vi "Edge Focus.vi"(8 "error in":errorcluster, 9 "Increment Size":dbl=-0.1 format="%#_13g", 10 "Position In":dbl=1.0 format="%#_13g", 11 "Gantry In":refnum<k24>) -> (0 "error out":errorcluster, 3 "Gantry Out":refnum<k24>)   [LabVIEW 2021, in "Component Tray.lvclass"]
uses:
  Component/Component Tray.lvclass
  C:/Program Files (x86)/Aerotech/A3200/LabVIEW/2010/Bin/Aerotech.A3200.dll
  Program Files (x86)/Aerotech/A3200/LabVIEW/2010/Bin/Aerotech.A3200.dll
  Controller/Motion/A3200/A3200.lvclass
  <vilib>/Analysis/NI_AALBase.lvlib
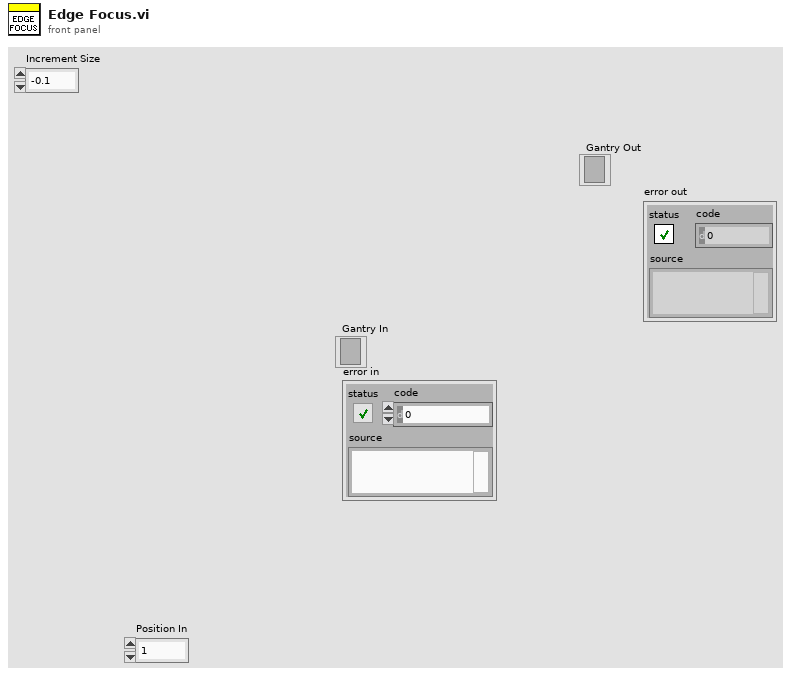
[diagram p1: front panel]
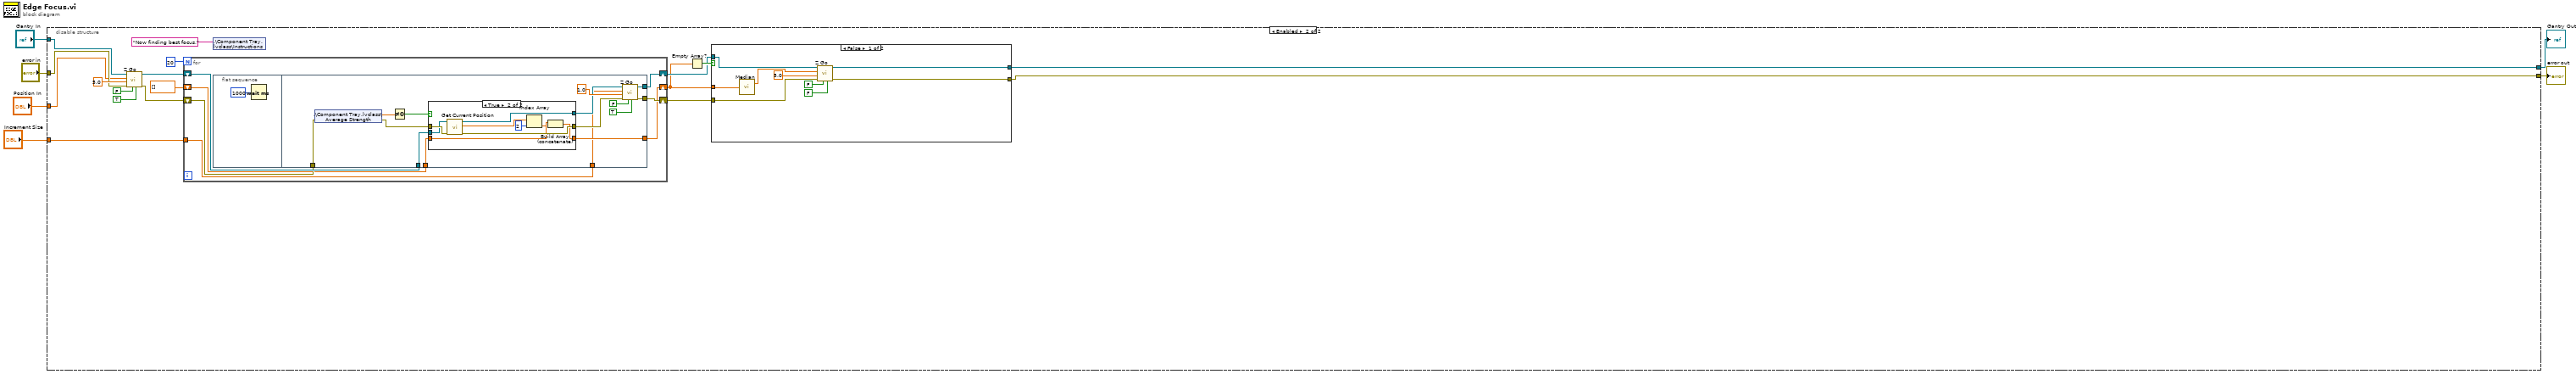
[diagram p0: block diagram]
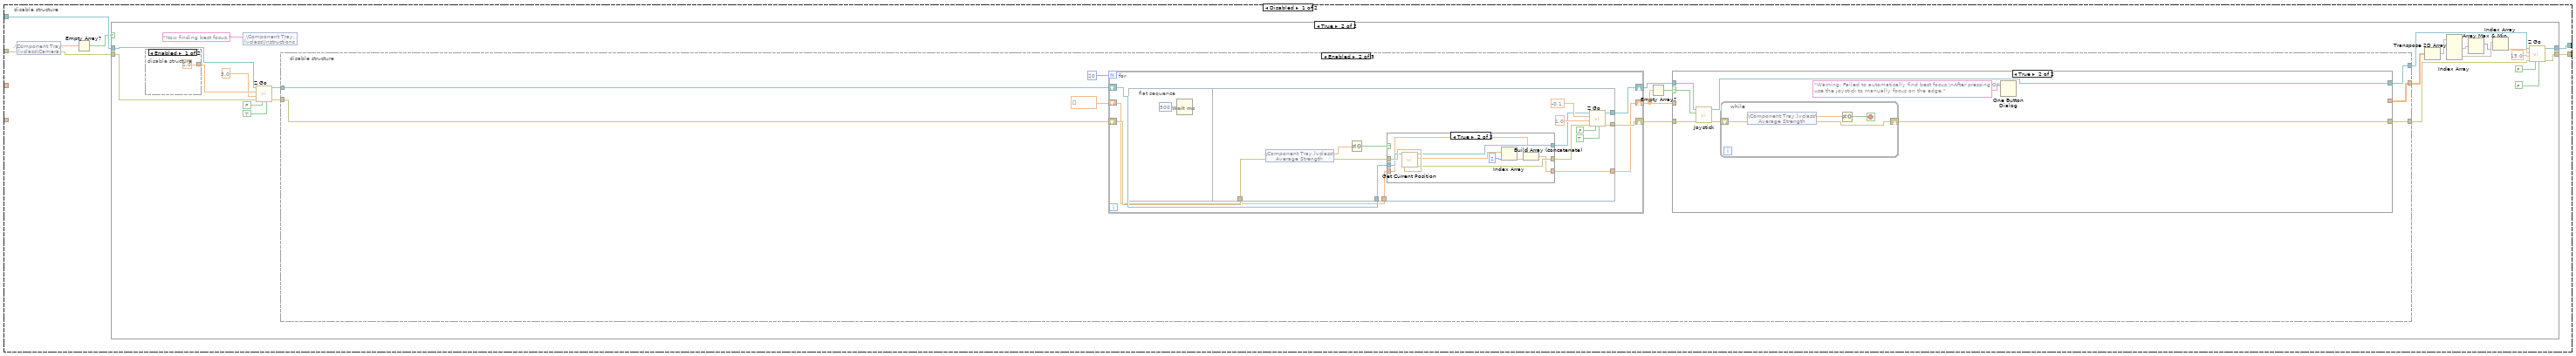
[diagram p2: hidden frame]
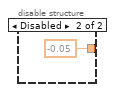
[diagram p4: hidden frame]
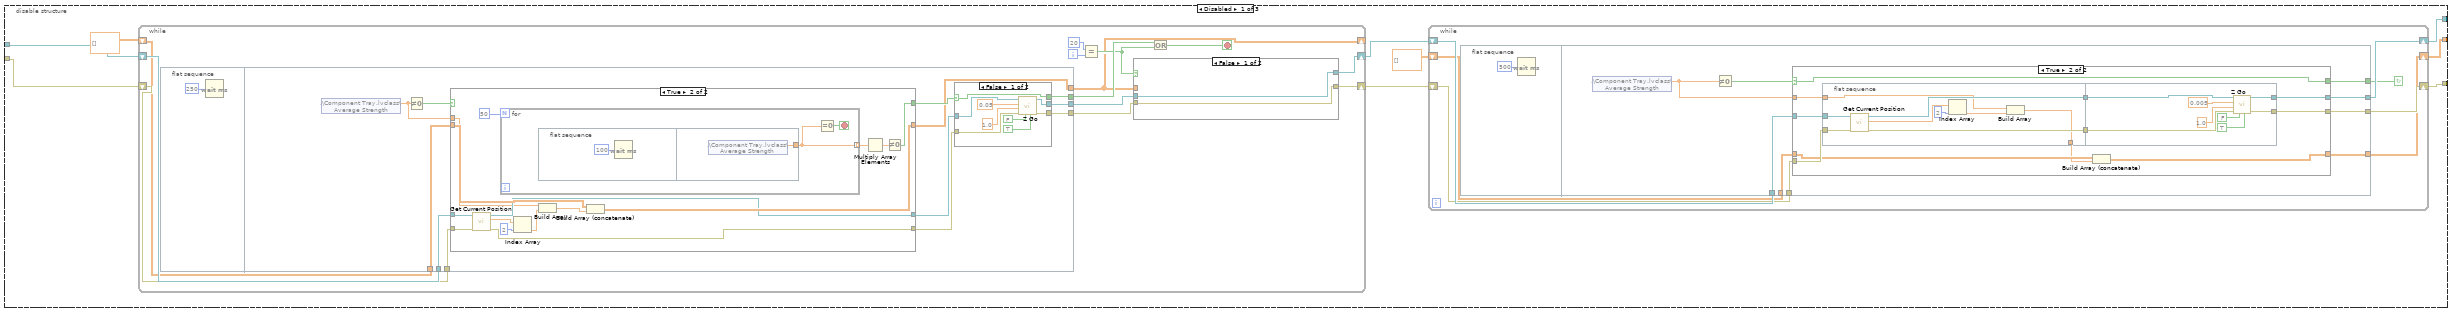
[diagram p5: hidden frame]
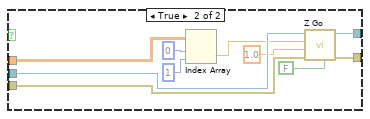
[diagram p6: hidden frame]
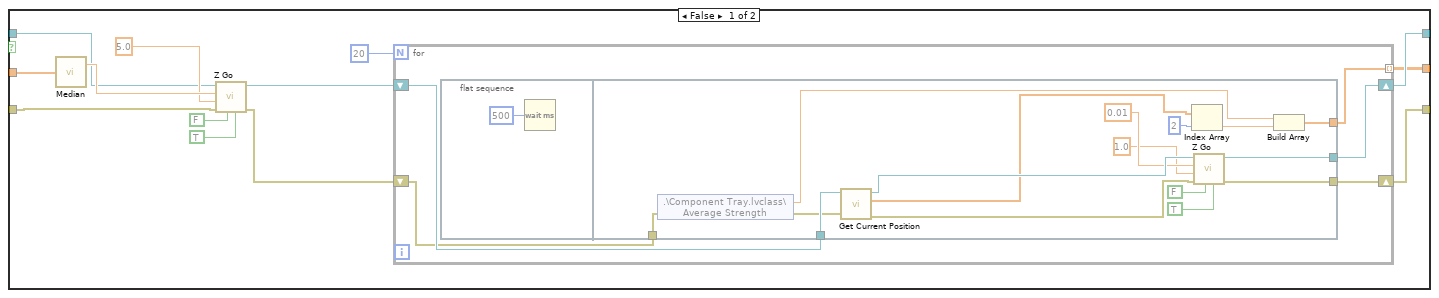
[diagram p10: hidden frame]
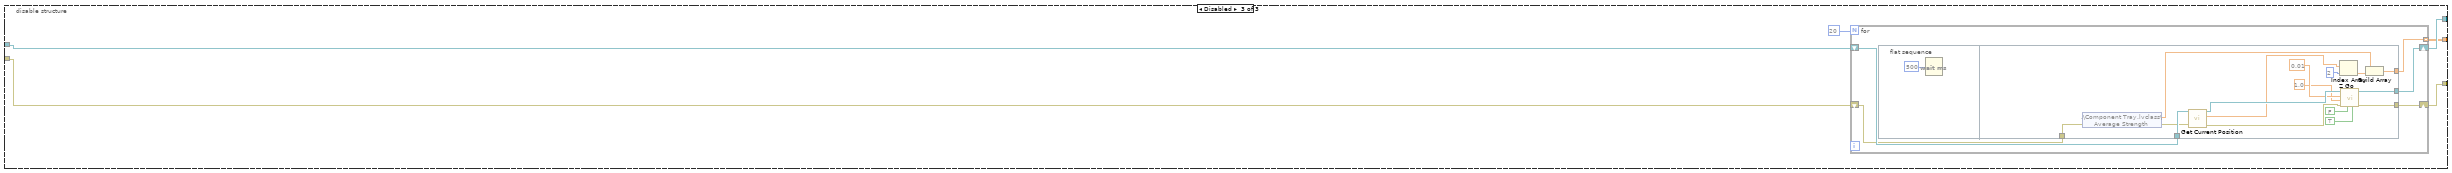
[diagram p12: hidden frame]
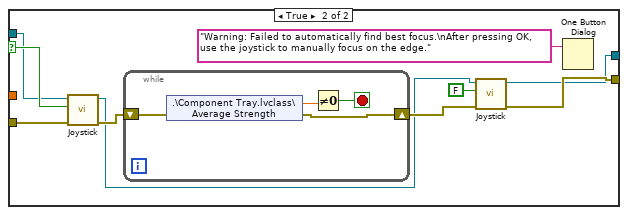
[diagram p13: hidden frame]
diagram:
  n1 = disable-structure shown="Enabled" {
    disable-tunnel: "Gantry In" -> [w13 w303]
    disable-tunnel: "error in" -> [w12 w300]
    disable-tunnel: [w11 w292] -> w4
    disable-tunnel: [w10 w291] -> w3
    disable-tunnel: "Position In" -> [_ w299]
    disable-tunnel: "Increment Size" -> [_ w296]
    frame Disabled {
      n2 = shared-variable ".\\Component Tray.lvclass\\Camera"(error in=w12) -> (w8:dbl[], error out=w9:errorcluster)
      n3 = Empty Array?(array=w8) -> (empty?=w7:bool)
      n4 = case shown="True" w7 {
        tunnel: w13 -> [w15 w26]
        tunnel: [w15 w24] -> w11
        tunnel: [w14 w23] -> w10
        tunnel: w9 -> [w14 w25]
        frame False {
        }
        frame True {
          n5 = disable-structure shown="Enabled" {
            disable-tunnel: [1.0 ("Position In") -0.05 ("Position In")] -> w21
            frame Enabled {
            }
            frame Disabled {
            }
          }
          n6 = shared-variable ".\\Component Tray.lvclass\\Instructions"("Now finding best focus." ("Instructions")) -> ()  [unwired: 1 in, 1 out]
          n7 = call "Z Go.vi"("Increment"=TRUE, "Return Immediately"=FALSE, "error in (no error)"=w25, "Speed In"=5.0, "Position In"=w21, "Gantry In"=w26) -> ("error out"=w16:errorcluster, "Gantry Out"=w17:refnum<k24>)  [unwired: 2 in, 2 out]
          n8 = disable-structure shown="Enabled" {
            disable-tunnel: [w48 w172 w264] -> w37
            disable-tunnel: [w47 w173 w267] -> w34
            disable-tunnel: [w46 w171 w265] -> w33
            disable-tunnel: w17 -> [w45 w181 w263]
            disable-tunnel: w16 -> [w44 w180 w266]
            frame Disabled {
              n9 = while {
                shift-right: [w52] -> w43
                shift-left: w45 -> [w61]
                shift-right: [w50] -> w42
                shift-left: w44 -> [w60]
                shift-right: [w51] -> _
                shift-left: dbl[][] [] ("Double") -> [w59]
                i -> [w58]
                stop <- w55 stop-if-true
                n10 = flat-sequence {
                  tunnel: w61 -> [w86]
                  tunnel: [w81] -> w53
                  tunnel: w60 -> [w85]
                  tunnel: [w80] -> w49
                  tunnel: [w83] -> w56
                  tunnel: [w75] -> w51
                  tunnel: w59 -> [w77]
                  frame #0 {
                    n11 = Wait (ms)(milliseconds to wait=u32 250) -> ()  [unwired: 1 out]
                  }
                  frame #1 {
                    n12 = shared-variable ".\\Component Tray.lvclass\\Average Strength"() -> (w76:dbl)  [unwired: 1 in, 1 out]
                    n13 = Not Equal To 0?(x=w76) -> (x != 0?=w78:bool)
                    n14 = case shown="True" w78 {
                      selector: w78 -> [w100 _]
                      tunnel: w86 -> [w102 w111]
                      tunnel: [w102 w110] -> w82
                      tunnel: w85 -> [w101 w109]
                      tunnel: [w101 w108] -> w79
                      tunnel: [w100 w114] -> w84
                      tunnel: w77 -> [w99 w113]
                      tunnel: w76 -> [_ w105]
                      tunnel: [w99 w112] -> w75
                      frame False {
                      }
                      frame True {
                        n15 = call "Get Current Position.vi"("error in (no error)"=w109, "Gantry In"=w111) -> ("error out"=w108:errorcluster, "XYZTheta Out"=w107:dbl[], "Gantry Out"=w110:refnum<k24>)  [unwired: 7 in]
                        n16 = for {
                          N: 50 -> [_]
                          tunnel: [w119] -> w116 mode=indexing
                          stop <- w118 stop-if-true
                          n17 = flat-sequence {
                            tunnel: [w121] -> w119
                            frame #0 {
                              n18 = Wait (ms)(milliseconds to wait=u32 100) -> ()  [unwired: 1 out]
                            }
                            frame #1 {
                              n19 = shared-variable ".\\Component Tray.lvclass\\Average Strength"() -> (w121:dbl)  [unwired: 1 in, 1 out]
                            }
                          }
                          n20 = Equal To 0?(x=w119) -> (x = 0?=w118:bool)
                        }
                        n21 = Index Array(array=w107, index=2) -> (element=w104:dbl)
                        n22 = Build Array(w105, w104) -> (w103:dbl[])
                        n23 = Build Array (concatenate)(w113, w103) -> (w112:dbl[][])
                        n24 = Multiply Array Elements(1:w116) -> (0:w115:dbl)
                        n25 = Not Equal To 0?(x=w115) -> (x != 0?=w114:bool)
                      }
                    }
                    n26 = case shown="False" w84 {
                      selector: w84 -> [w91 w98]
                      tunnel: [w91 w98] -> w83
                      tunnel: w82 -> [w90 w97]
                      tunnel: [w89 w97] -> w81
                      tunnel: [w88 w96] -> w80
                      tunnel: w79 -> [w87 w96]
                      frame False {
                        n27 = call "Z Go.vi"("Increment"=TRUE, "Return Immediately"=FALSE, "error in (no error)"=w87, "Speed In"=1.0, "Position In"=0.05, "Gantry In"=w90) -> ("error out"=w88:errorcluster, "Gantry Out"=w89:refnum<k24>)  [unwired: 2 in, 2 out]
                      }
                      frame True {
                      }
                    }
                  }
                }
                n28 = Equal?(x=20, y=w58) -> (x = y?=w54:bool)
                n29 = case shown="False" w54 {
                  tunnel: w53 -> [w63 w73]
                  tunnel: [w63 w72] -> w52
                  tunnel: w51 -> [_ w71]
                  tunnel: [w62 w66] -> w50
                  tunnel: w49 -> [w62 w65]
                  frame False {
                  }
                  frame True {
                    n30 = Index Array(array=w71, index (row)=0, index (col)=1 ("disabled index (col)")) -> (element=w68:dbl)
                    n31 = call "Z Go.vi"("Increment"=FALSE, "error in (no error)"=w65, "Speed In"=1.0, "Position In"=w68, "Gantry In"=w73) -> ("error out"=w66:errorcluster, "Gantry Out"=w72:refnum<k24>)  [unwired: 3 in, 2 out]
                  }
                }
                n32 = Or(x=w56, y=w54) -> (x .or. y?=w55:bool)
              }
              n33 = while {
                shift-right: [w127] -> w47
                shift-left: w43 -> [w128]
                shift-right: [w125] -> w46
                shift-left: w42 -> [w126]
                shift-right: [w122] -> w48
                shift-left: dbl[][] [] -> [w123]
                stop <- w124 continue-if-true
                n34 = flat-sequence {
                  tunnel: w128 -> [w138]
                  tunnel: [w135] -> w127
                  tunnel: w126 -> [w137]
                  tunnel: [w134] -> w125
                  tunnel: [w136] -> w124
                  tunnel: [w133] -> w122
                  tunnel: w123 -> [w132]
                  frame #0 {
                    n35 = Wait (ms)(milliseconds to wait=u32 500) -> ()  [unwired: 1 out]
                  }
                  frame #1 {
                    n36 = shared-variable ".\\Component Tray.lvclass\\Average Strength"() -> (w130:dbl)  [unwired: 1 in, 1 out]
                    n37 = Not Equal To 0?(x=w130) -> (x != 0?=w131:bool)
                    n38 = case shown="True" w131 {
                      selector: w131 -> [w142 w153]
                      tunnel: [w142 w153] -> w136
                      tunnel: w138 -> [w141 w152]
                      tunnel: [w141 w151] -> w135
                      tunnel: [w140 w150] -> w134
                      tunnel: w137 -> [w140 w149]
                      tunnel: [w139 w144] -> w133
                      tunnel: w132 -> [w139 w146]
                      tunnel: w130 -> [_ w143]
                      frame False {
                      }
                      frame True {
                        n39 = flat-sequence {
                          tunnel: w149 -> [w156]
                          tunnel: w152 -> [w158]
                          tunnel: [w157] -> w148
                          tunnel: [w159] -> w147
                          tunnel: [w155] -> w145
                          tunnel: w143 -> [w154]
                          tunnel: [w165] -> w151
                          tunnel: [w164] -> w150
                          tunnel: w148 -> [w166]
                          tunnel: w147 -> [w163]
                          frame #0 {
                            n40 = call "Get Current Position.vi"("error in (no error)"=w156, "Gantry In"=w158) -> ("error out"=w159:errorcluster, "XYZTheta Out"=w162:dbl[], "Gantry Out"=w157:refnum<k24>)  [unwired: 7 in]
                            n41 = Index Array(array=w162, index=2) -> (element=w160:dbl)
                            n42 = Build Array(w154, w160) -> (w155:dbl[])
                          }
                          frame #1 {
                            n43 = call "Z Go.vi"("Increment"=TRUE, "Return Immediately"=FALSE, "error in (no error)"=w163, "Speed In"=1.0, "Position In"=0.005, "Gantry In"=w166) -> ("error out"=w164:errorcluster, "Gantry Out"=w165:refnum<k24>)  [unwired: 2 in, 2 out]
                          }
                        }
                        n44 = Build Array (concatenate)(w146, w145) -> (w144:dbl[][])
                      }
                    }
                  }
                }
              }
            }
            frame Enabled {
              n45 = for {
                N: 20 -> [_]
                shift-right: [w232] -> w175
                shift-left: w181 -> [w233]
                shift-right: [w230] -> w176
                shift-left: w180 -> [w231]
                shift-right: [w229] -> w174
                shift-left: dbl[] [] -> [w228]
                n46 = flat-sequence {
                  tunnel: [w249] -> w232
                  tunnel: [w248] -> w230
                  tunnel: [w236] -> w229
                  tunnel: w233 -> [w240]
                  tunnel: w231 -> [w243]
                  tunnel: w228 -> [w235]
                  frame #0 {
                    n47 = Wait (ms)(milliseconds to wait=u32 500) -> ()  [unwired: 1 out]
                  }
                  frame #1 {
                    n48 = shared-variable ".\\Component Tray.lvclass\\Average Strength"(error in=w243) -> (w237:dbl, error out=w241:errorcluster)
                    n49 = Not Equal To 0?(x=w237) -> (x != 0?=w242:bool)
                    n50 = case shown="True" w242 {
                      tunnel: w241 -> [w251 w261]
                      tunnel: w240 -> [w252 w260]
                      tunnel: [w251 w259] -> w239
                      tunnel: [w252 w258] -> w238
                      tunnel: [w250 w254] -> w236
                      tunnel: w235 -> [w250 w255]
                      frame False {
                      }
                      frame True {
                        n51 = call "Get Current Position.vi"("error in (no error)"=w261, "Gantry In"=w260) -> ("error out"=w259:errorcluster, "XYZTheta Out"=w257:dbl[], "Gantry Out"=w258:refnum<k24>)  [unwired: 7 in]
                        n52 = Index Array(array=w257, index=2) -> (element=w253:dbl)
                        n53 = Build Array (concatenate)(w255, w253) -> (w254:dbl[])
                      }
                    }
                    n54 = call "Z Go.vi"("Increment"=TRUE, "Return Immediately"=FALSE, "error in (no error)"=w239, "Speed In"=1.0, "Position In"=-0.1, "Gantry In"=w238) -> ("error out"=w248:errorcluster, "Gantry Out"=w249:refnum<k24>)  [unwired: 2 in, 2 out]
                  }
                }
              }
              n55 = Empty Array?(array=w174) -> (empty?=w177:bool)
              n56 = case shown="True" w177 {
                selector: w177 -> [_ w222]
                tunnel: w176 -> [w191 w221]
                tunnel: w175 -> [w189 w223]
                tunnel: w174 -> [w188 _]
                tunnel: [w184 w218] -> w173
                tunnel: [w183 _] -> w172
                tunnel: [w182 w217] -> w171
                frame False {
                  n57 = call <vilib>:"Median.vi"("X"=w188) -> ("median"=w194:dbl)  [unwired: 1 out]
                  n58 = call "Z Go.vi"("Increment"=TRUE, "Return Immediately"=FALSE, "error in (no error)"=w191, "Speed In"=5.0, "Position In"=w194, "Gantry In"=w189) -> ("error out"=w185:errorcluster, "Gantry Out"=w186:refnum<k24>)  [unwired: 2 in, 2 out]
                  n59 = for {
                    N: 20 -> [_]
                    shift-right: [w198] -> w184
                    shift-left: w186 -> [w199]
                    tunnel: [w195] -> w183 mode=indexing
                    shift-right: [w196] -> w182
                    shift-left: w185 -> [w197]
                    n60 = flat-sequence {
                      tunnel: [w216] -> w198
                      tunnel: [w215] -> w196
                      tunnel: [w211] -> w195
                      tunnel: w199 -> [w214]
                      tunnel: w197 -> [w201]
                      frame #0 {
                        n61 = Wait (ms)(milliseconds to wait=u32 500) -> ()  [unwired: 1 out]
                      }
                      frame #1 {
                        n62 = shared-variable ".\\Component Tray.lvclass\\Average Strength"(error in=w201) -> (w202:dbl, error out=w203:errorcluster)
                        n63 = call "Get Current Position.vi"("error in (no error)"=w203, "Gantry In"=w214) -> ("error out"=w212:errorcluster, "XYZTheta Out"=w210:dbl[], "Gantry Out"=w213:refnum<k24>)  [unwired: 7 in]
                        n64 = Index Array(array=w210, index=2) -> (element=w208:dbl)
                        n65 = call "Z Go.vi"("Increment"=TRUE, "Return Immediately"=FALSE, "error in (no error)"=w212, "Speed In"=1.0, "Position In"=0.01, "Gantry In"=w213) -> ("error out"=w215:errorcluster, "Gantry Out"=w216:refnum<k24>)  [unwired: 2 in, 2 out]
                        n66 = Build Array(w202, w208) -> (w211:dbl[])
                      }
                    }
                  }
                }
                frame True {
                  n67 = call "Joystick.vi"("error in (no error)"=w221, "Joystick"=w222, "Gantry In"=w223) -> ("error out"=w219:errorcluster, "Gantry Out"=w218:refnum<k24>)  [unwired: 7 in]
                  n68 = while {
                    shift-right: [w224] -> w217
                    shift-left: w219 -> [w225]
                    stop <- w226 stop-if-true
                    n69 = shared-variable ".\\Component Tray.lvclass\\Average Strength"(error in=w225) -> (w227:dbl, error out=w224:errorcluster)
                    n70 = Not Equal To 0?(x=w227) -> (x != 0?=w226:bool)
                  }
                  n71 = One Button Dialog(message="Warning: Failed to automatically find best focus.\nAfter pressing OK, use the joystick to manually focus on the edge.") -> ()  [unwired: 1 in, 1 out]
                }
              }
            }
            frame Disabled {
              n72 = for {
                N: 20 -> [_]
                shift-right: [w271] -> w267
                shift-left: w263 -> [w272]
                tunnel: [w268] -> w264 mode=indexing
                shift-right: [w269] -> w265
                shift-left: w266 -> [w270]
                n73 = flat-sequence {
                  tunnel: [w289] -> w271
                  tunnel: [w288] -> w269
                  tunnel: [w284] -> w268
                  tunnel: w272 -> [w287]
                  tunnel: w270 -> [w274]
                  frame #0 {
                    n74 = Wait (ms)(milliseconds to wait=u32 500) -> ()  [unwired: 1 out]
                  }
                  frame #1 {
                    n75 = shared-variable ".\\Component Tray.lvclass\\Average Strength"(error in=w274) -> (w275:dbl, error out=w276:errorcluster)
                    n76 = call "Get Current Position.vi"("error in (no error)"=w276, "Gantry In"=w287) -> ("error out"=w285:errorcluster, "XYZTheta Out"=w283:dbl[], "Gantry Out"=w286:refnum<k24>)  [unwired: 7 in]
                    n77 = Index Array(array=w283, index=2) -> (element=w281:dbl)
                    n78 = call "Z Go.vi"("Increment"=TRUE, "Return Immediately"=FALSE, "error in (no error)"=w285, "Speed In"=1.0, "Position In"=0.01, "Gantry In"=w286) -> ("error out"=w288:errorcluster, "Gantry Out"=w289:refnum<k24>)  [unwired: 2 in, 2 out]
                    n79 = Build Array(w275, w281) -> (w284:dbl[])
                  }
                }
              }
            }
          }
          n80 = Transpose 2D Array(2D array=w37) -> (transposed array=w30:dbl[][])
          n81 = Index Array(array=w30) -> (element #1=w27:dbl[], element #2=w29:dbl[])  [unwired: 4 in]
          n82 = Array Max & Min(array=w27) -> (max index (indices)=w28:i32)  [unwired: 3 out]
          n83 = Index Array(array=w29, index=w28) -> (element=w36:dbl)
          n84 = call "Z Go.vi"("Increment"=FALSE, "Return Immediately"=FALSE ("Increment"), "error in (no error)"=w33, "Speed In"=15.0 ("Speed"), "Position In"=w36, "Gantry In"=w34) -> ("error out"=w23:errorcluster, "Gantry Out"=w24:refnum<k24>)  [unwired: 2 in, 2 out]
        }
      }
    }
    frame Enabled {
      n85 = call "Z Go.vi"("Increment"=TRUE, "Return Immediately"=FALSE, "error in (no error)"=w300, "Speed In"=5.0, "Position In"=w299, "Gantry In"=w303) -> ("error out"=w301:errorcluster, "Gantry Out"=w302:refnum<k24>)  [unwired: 2 in, 2 out]
      n86 = for {
        N: 20 -> [_]
        shift-right: [w336] -> w293
        shift-left: w302 -> [w337]
        shift-right: [w334] -> w294
        shift-left: w301 -> [w335]
        shift-right: [w333] -> w290
        shift-left: dbl[] [] -> [w332]
        tunnel: w296 -> [w331]
        n87 = flat-sequence {
          tunnel: [w353] -> w336
          tunnel: [w352] -> w334
          tunnel: [w341] -> w333
          tunnel: w337 -> [w345]
          tunnel: w335 -> [w348]
          tunnel: w332 -> [w340]
          tunnel: w331 -> [w339]
          frame #0 {
            n88 = Wait (ms)(milliseconds to wait=u32 1000) -> ()  [unwired: 1 out]
          }
          frame #1 {
            n89 = shared-variable ".\\Component Tray.lvclass\\Average Strength"(error in=w348) -> (w342:dbl, error out=w346:errorcluster)
            n90 = Not Equal To 0?(x=w342) -> (x != 0?=w347:bool)
            n91 = case shown="True" w347 {
              tunnel: w346 -> [w355 w365]
              tunnel: w345 -> [w356 w364]
              tunnel: [w355 w363] -> w344
              tunnel: [w356 w362] -> w343
              tunnel: [w354 w358] -> w341
              tunnel: w340 -> [w354 w359]
              frame False {
              }
              frame True {
                n92 = call "Get Current Position.vi"("error in (no error)"=w365, "Gantry In"=w364) -> ("error out"=w363:errorcluster, "XYZTheta Out"=w361:dbl[], "Gantry Out"=w362:refnum<k24>)  [unwired: 7 in]
                n93 = Index Array(array=w361, index=2) -> (element=w357:dbl)
                n94 = Build Array (concatenate)(w359, w357) -> (w358:dbl[])
              }
            }
            n95 = call "Z Go.vi"("Increment"=TRUE, "Return Immediately"=FALSE, "error in (no error)"=w344, "Speed In"=1.0, "Position In"=w339, "Gantry In"=w343) -> ("error out"=w352:errorcluster, "Gantry Out"=w353:refnum<k24>)  [unwired: 2 in, 2 out]
          }
        }
      }
      n96 = shared-variable ".\\Component Tray.lvclass\\Instructions"("Now finding best focus." ("Instructions")) -> ()  [unwired: 1 in, 1 out]
      n97 = Empty Array?(array=w290) -> (empty?=w295:bool)
      n98 = case shown="False" w295 {
        selector: w295 -> [_ w326]
        tunnel: [w309 w320] -> w292
        tunnel: [w308 w322] -> w291
        tunnel: w294 -> [w310 w318]
        tunnel: w293 -> [w312 w317]
        tunnel: w290 -> [w311 _]
        frame False {
          n99 = call <vilib>:"Median.vi"("X"=w311) -> ("median"=w313:dbl)  [unwired: 1 out]
          n100 = call "Z Go.vi"("Increment"=FALSE, "Return Immediately"=FALSE, "error in (no error)"=w310, "Speed In"=5.0, "Position In"=w313, "Gantry In"=w312) -> ("error out"=w308:errorcluster, "Gantry Out"=w309:refnum<k24>)  [unwired: 2 in, 2 out]
        }
        frame True {
          n101 = call "Joystick.vi"("error in (no error)"=w318, "Joystick"=w326, "Gantry In"=w317) -> ("error out"=w324:errorcluster, "Gantry Out"=w321:refnum<k24>)  [unwired: 7 in]
          n102 = while {
            shift-right: [w327] -> w323
            shift-left: w324 -> [w328]
            stop <- w329 stop-if-true
            n103 = shared-variable ".\\Component Tray.lvclass\\Average Strength"(error in=w328) -> (w330:dbl, error out=w327:errorcluster)
            n104 = Not Equal To 0?(x=w330) -> (x != 0?=w329:bool)
          }
          n105 = call "Joystick.vi"("error in (no error)"=w323, "Joystick"=FALSE, "Gantry In"=w321) -> ("error out"=w322:errorcluster, "Gantry Out"=w320:refnum<k24>)  [unwired: 7 in]
          n106 = One Button Dialog(message="Warning: Failed to automatically find best focus.\nAfter pressing OK, use the joystick to manually focus on the edge.") -> ()  [unwired: 1 in, 1 out]
        }
      }
    }
  }
  "Gantry Out" <- w4
  "error out" <- w3
